vi "I.vi"(1 "Promien krzywizny południka [v]":ext, 2 "t":ext, 3 "fi[rad]":ext) -> (0 "D":ext)   [LabVIEW 2015, in "Biblioteka moduł map v3.lvlib" / "Konwersja wsp.lvlib" / "UTM.lvlib" / "Konwersja na UTM.lvlib"]
doc: "Współczynnik wzoru na konwersję na UTM."
uses:
  Konwersja na UTM.lvlib
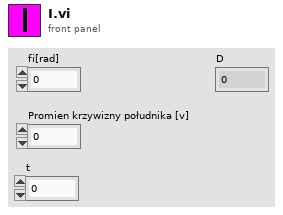
[diagram p1: front panel]
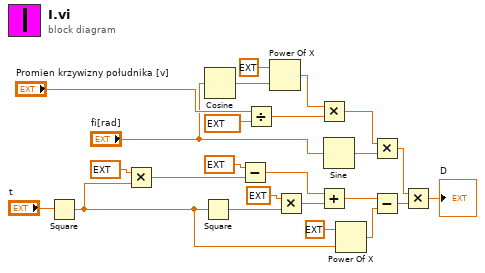
[diagram p0: block diagram]
diagram:
  n1 = Square(x="t") -> (x^2=w8:ext)
  n2 = Multiply(x=ext 3111.0 ("y"), y=w8) -> (x*y=w14:ext)
  n3 = Square(x=w8) -> (x^2=w9:ext)
  n4 = Cosine(x="fi[rad]") -> (cos(x)=w20:ext)
  n5 = Subtract(x=ext 1385.0 ("y"), y=w14) -> (x-y=w13:ext)
  n6 = Divide(x="Promien krzywizny południka [v]", y=ext 40320.0) -> (x/y=w23:ext)
  n7 = Power Of X(1:w20, 2:ext 7.0 ("y")) -> (0:w22:ext)
  n8 = Multiply(x=ext 543.0 ("y"), y=w9) -> (x*y=w11:ext)
  n9 = Multiply(x=w22, y=w23) -> (x*y=w4:ext)
  n10 = Add(x=w13, y=w11) -> (x+y=w10:ext)
  n11 = Sine(x="fi[rad]") -> (sin(x)=w2:ext)
  n12 = Power Of X(1:w8, 2:ext 3.0 ("y")) -> (0:w6:ext)
  n13 = Multiply(x=w4, y=w2) -> (x*y=w1:ext)
  n14 = Subtract(x=w10, y=w6) -> (x-y=w5:ext)
  n15 = Multiply(x=w1, y=w5) -> (x*y=→"D":ext)
